vi "Receiver.vi"() -> (0 "Channel 7 position":i32, 1 "Channel 6 position":i32, 2 "Channel 5 position":i32, 3 "Channel 4 position":i32)   [LabVIEW 2016]
doc: "Inputs\n-\n\nOutputs\nPosition for channel 4, 5, 6, 7\nValue channel 0\n\nThis VI reads the signals from the RC receiver, process the data and outputs the position on the switches (channel 4. 5, 6, 7) and the value for channel 0 which corresponds to the horisontal positon of the right joystick."
uses:
  <vilib>/eio/EIONode/EIONode.xnode
  <vilib>/rvi/eio/common/nirviEmuTemplateMethod_errors.vi
panel:
  in  "Sync Pulse Max":u32=15000
  in  "Sync Pulse Min":u32=3500
  out "Value Channel 3":u32
  out "Value Channel 2":u32
  out "Value Channel 1":u32
  out "Value Channel 0":u32
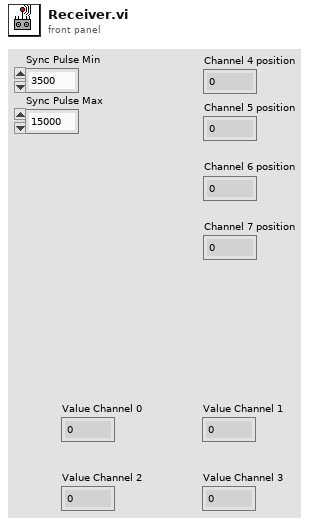
[diagram p1: front panel]
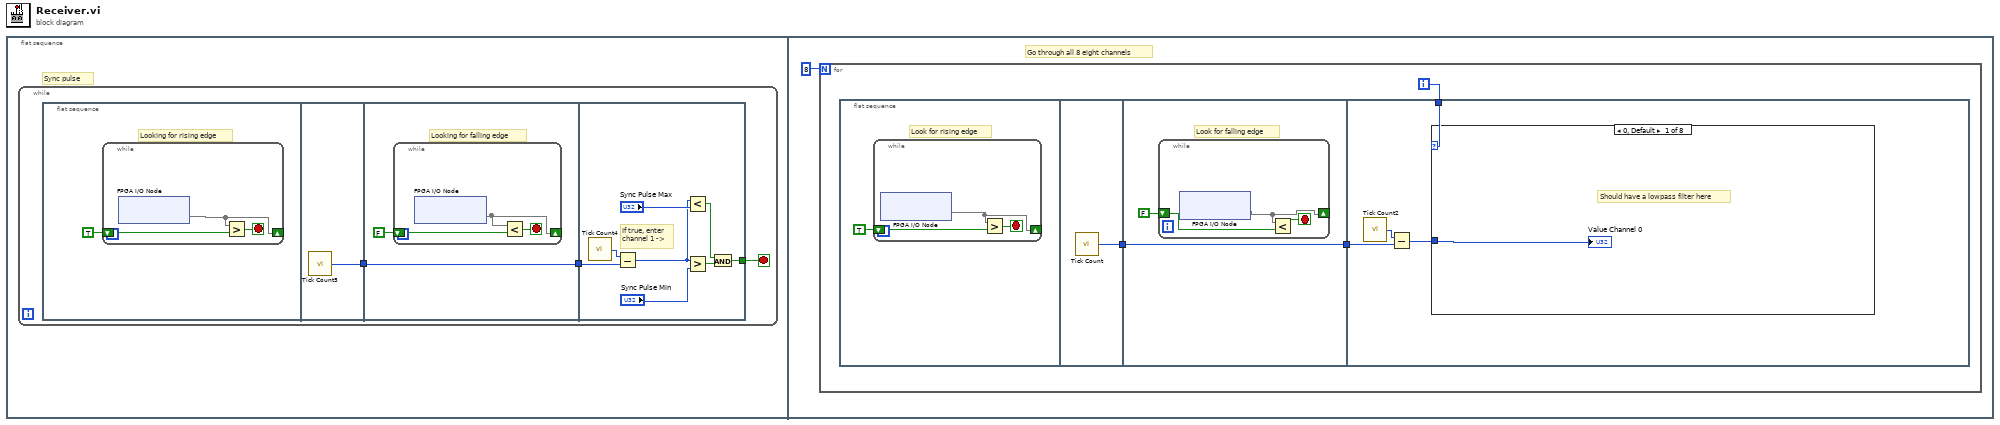
[diagram p0: block diagram]
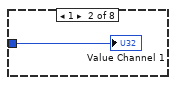
[diagram p2: hidden frame]
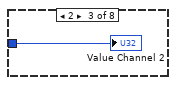
[diagram p3: hidden frame]
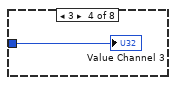
[diagram p4: hidden frame]
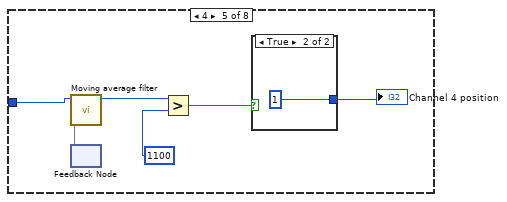
[diagram p5: hidden frame]
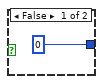
[diagram p6: hidden frame]
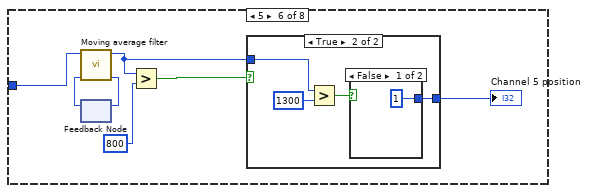
[diagram p7: hidden frame]
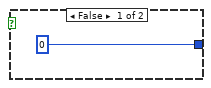
[diagram p8: hidden frame]
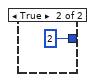
[diagram p9: hidden frame]
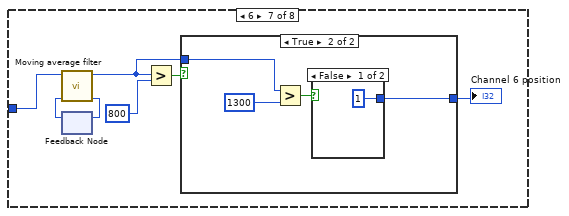
[diagram p10: hidden frame]
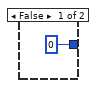
[diagram p11: hidden frame]
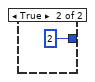
[diagram p12: hidden frame]
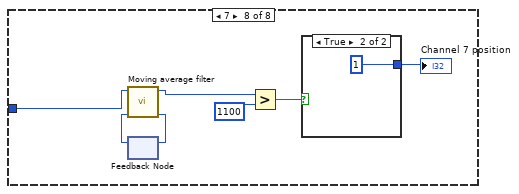
[diagram p13: hidden frame]
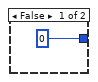
[diagram p14: hidden frame]
diagram:
  n1 = flat-sequence {
    frame #0 {
      # "Sync pulse"
      n2 = while {
        stop <- w1 stop-if-true
        n3 = flat-sequence {
          tunnel: [w8] -> w3
          tunnel: w3 -> [w9]
          tunnel: [w9] -> w2
          tunnel: [w21] -> w1
          tunnel: w2 -> [w16]
          frame #0 {
            # "Looking for rising edge"
            n4 = while {
              shift-right: [w5] -> _
              shift-left: TRUE -> [w6]
              stop <- w7 stop-if-true
              n5 = xnode "FPGA I/O Node"() -> ("DIO/DIO4"=w5)  [unwired: 1 in, 1 out]
              n6 = Greater?(x=w5, y=w6) -> (0:w7:bool)
            }
          }
          frame #1 {
            n7 = call "Tick Count5"() -> ("Tick Count(uSec)"=w8:u32)
          }
          frame #2 {
            # "Looking for falling edge"
            n8 = while {
              shift-right: [w11] -> _
              shift-left: FALSE -> [w12]
              stop <- w13 stop-if-true
              n9 = xnode "FPGA I/O Node"() -> ("DIO/DIO4"=w11)  [unwired: 1 in, 1 out]
              n10 = Less?(x=w11, y=w12) -> (x < y?=w13:bool)
            }
          }
          frame #3 {
            # "If true, enter \nchannel 1 ->"
            n11 = call "Tick Count4"() -> ("Tick Count(uSec)"=w17:u32)
            n12 = Subtract(x=w17, y=w16) -> (x-y=w14:u32)
            n13 = Less?(x=w14, y="Sync Pulse Max") -> (x < y?=w19:bool)
            n14 = Greater?(x=w14, y="Sync Pulse Min") -> (0:w20:bool)
            n15 = And(x=w19, y=w20) -> (x .and. y?=w21:bool)
          }
        }
      }
    }
    frame #1 {
      # "Go through all 8 eight channels"
      n16 = for {
        N: 8 -> [_]
        i -> [w23]
        n17 = flat-sequence {
          tunnel: [w30] -> w25
          tunnel: [w31] -> w24
          tunnel: w25 -> [w31]
          tunnel: w23 -> [w39]
          tunnel: w24 -> [w37]
          frame #0 {
            # "Look for rising edge"
            n18 = while {
              shift-right: [w27] -> _
              shift-left: TRUE -> [w28]
              stop <- w29 stop-if-true
              n19 = xnode "FPGA I/O Node"() -> ("DIO/DIO4"=w27)  [unwired: 1 in, 1 out]
              n20 = Greater?(x=w27, y=w28) -> (0:w29:bool)
            }
          }
          frame #1 {
            n21 = call "Tick Count"() -> ("Tick Count(uSec)"=w30:u32)
          }
          frame #2 {
            # "Look for falling edge"
            n22 = while {
              shift-right: [w33] -> _
              shift-left: FALSE -> [w34]
              stop <- w35 stop-if-true
              n23 = xnode "FPGA I/O Node"() -> ("DIO/DIO4"=w33)  [unwired: 1 in, 1 out]
              n24 = Less?(x=w33, y=w34) -> (x < y?=w35:bool)
            }
          }
          frame #3 {
            n25 = call "Tick Count2"() -> ("Tick Count(uSec)"=w38:u32)
            n26 = Subtract(x=w38, y=w37) -> (x-y=w36:u32)
            n27 = case shown="0, Default" w39 {
              tunnel: w36 -> [w40 w41 w42 w43 w45 w53 w67 w82]
              frame 0, Default {
                # "Should have a lowpass filter here"
                "Value Channel 0" <- w40
              }
              frame 1 {
                "Value Channel 1" <- w41
              }
              frame 2 {
                "Value Channel 2" <- w42
              }
              frame 3 {
                "Value Channel 3" <- w43
              }
              frame 4 {
                n28 = feedback #1() -> (w44)  [unwired: 1 in]
                n29 = call "Moving average filter.vi"("x"=w44, "Input"=w45) -> ("Mean"=w46:i32)  [unwired: 8 in, 1 out]
                n30 = feedback-in #1() -> ()  [unwired: 1 out]
                n31 = Greater?(x=w46, y=u32 1100) -> (0:w48:bool)
                n32 = case shown="True" w48 {
                  tunnel: [0 1] -> w47
                  frame False {
                  }
                  frame True {
                  }
                }
                "Channel 4 position" <- w47
              }
              frame 5 {
                n33 = feedback #2() -> (w56:i32)  [unwired: 1 in]
                n34 = call "Moving average filter.vi"("x"=w56, "Input"=w53) -> ("xdot"=w55:i32, "Mean"=w54:i32)  [unwired: 8 in]
                n35 = feedback-in #2(w55) -> ()
                n36 = Greater?(x=w54, y=800) -> (0:w58:bool)
                n37 = case shown="True" w58 {
                  tunnel: w54 -> [_ w62]
                  tunnel: [0 w60] -> w57
                  frame False {
                  }
                  frame True {
                    n38 = Greater?(x=w62, y=1300) -> (0:w63:bool)
                    n39 = case shown="False" w63 {
                      tunnel: [1 2] -> w60
                      frame False {
                      }
                      frame True {
                      }
                    }
                  }
                }
                "Channel 5 position" <- w57
              }
              frame 6 {
                n40 = feedback #3() -> (w69:i32)  [unwired: 1 in]
                n41 = call "Moving average filter.vi"("x"=w69, "Input"=w67) -> ("xdot"=w68:i32, "Mean"=w66:i32)  [unwired: 8 in]
                n42 = feedback-in #3(w68) -> ()
                n43 = Greater?(x=w66, y=800) -> (0:w71:bool)
                n44 = case shown="True" w71 {
                  tunnel: w66 -> [_ w76]
                  tunnel: [0 w75] -> w72
                  frame False {
                  }
                  frame True {
                    n45 = Greater?(x=w76, y=1300) -> (0:w77:bool)
                    n46 = case shown="False" w77 {
                      tunnel: [1 2] -> w75
                      frame False {
                      }
                      frame True {
                      }
                    }
                  }
                }
                "Channel 6 position" <- w72
              }
              frame 7 {
                n47 = feedback #4() -> (w81:i32)  [unwired: 1 in]
                n48 = call "Moving average filter.vi"("x"=w81, "Input"=w82) -> ("xdot"=w80:i32, "Mean"=w83:i32)  [unwired: 8 in]
                n49 = feedback-in #4(w80) -> ()
                n50 = Greater?(x=w83, y=1100) -> (0:w86:bool)
                n51 = case shown="True" w86 {
                  tunnel: [0 1] -> w84
                  frame False {
                  }
                  frame True {
                  }
                }
                "Channel 7 position" <- w84
              }
            }
          }
        }
      }
    }
  }
